vi "AddNamedRendezvousPrefix.vi"(10 "String In":string) -> (2 "String Out":string)   [LabVIEW 2010]
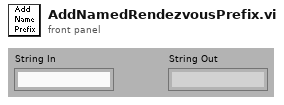
[diagram p1: front panel]
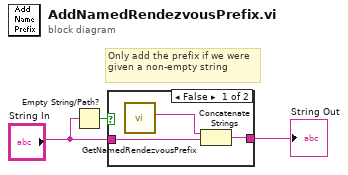
[diagram p0: block diagram]
diagram:
  # "Only add the prefix if we were given a non-empty string"
  n1 = Empty String/Path?(string/path="String In") -> (empty?=w3:bool)
  n2 = case shown="False" w3 {
    tunnel: "String In" -> [w6 w7]
    tunnel: [w5 w7] -> w1
    frame False {
      n3 = call "GetNamedRendezvousPrefix.vi"() -> ("Named Semaphore Prefix"=w4:string)  [unwired: 11 out]
      n4 = Concatenate Strings(w4, w6) -> (w5:string)
    }
    frame True {
    }
  }
  "String Out" <- w1
